vi "PH_Beckhoff-16BB.declare digital OutputTags.vi"(2 "Racktype":string, 3 "Digital Outputs to be inverted [#s separated by ::]":string, 4 "Instance Name":string="<Instance Name>") -> (0 "Digital Outputs":T1, 1 "Description":string)   [LabVIEW 2014, in "PH_Beckhoff-16BB.lvlib"]
uses:
  PH_Beckhoff-16BB.lvlib
  PH_Beckhoff/PH_Beckhoff.Digital Outputs.ctl
  PH_Beckhoff/PH_Beckhoff.lvlib
  PH_Beckhoff_Common/PH_Beckhoff_Common.lvlib
panel:
  out "Right Size?":bool
  # "Let this VI run to check the size!"
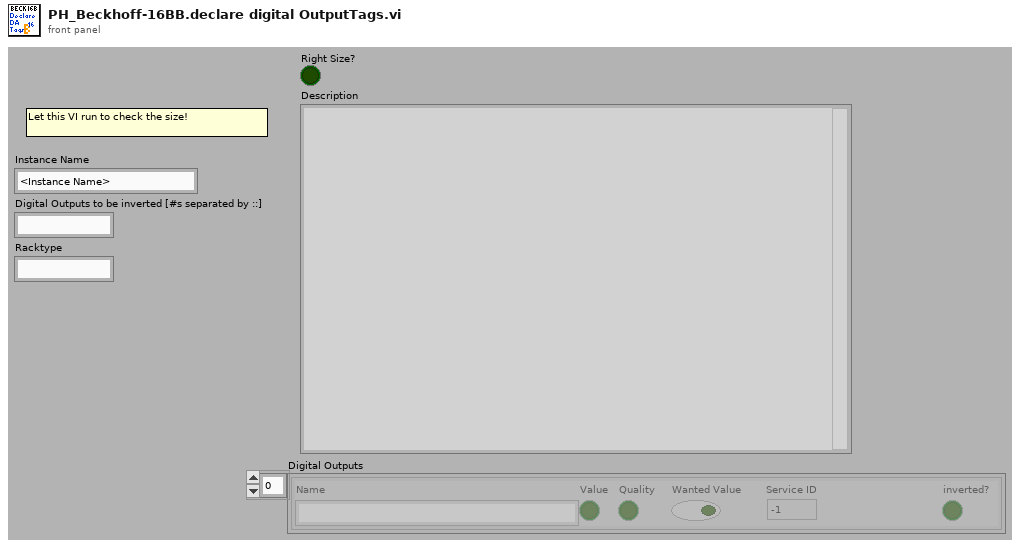
[diagram p1: front panel]
types:
  T1 = typedef "PH_Beckhoff.lvlib/PH_Beckhoff.Digital Outputs.ctl" = cluster{"Name":string, "Value":bool, "Quality":bool, "Wanted Value":bool, "Service ID":i32, "inverted?":bool}[]
  T2 = cluster{"Name":string, "Value":bool, "Quality":bool, "Wanted Value":bool, "Service ID":i32, "inverted?":bool}
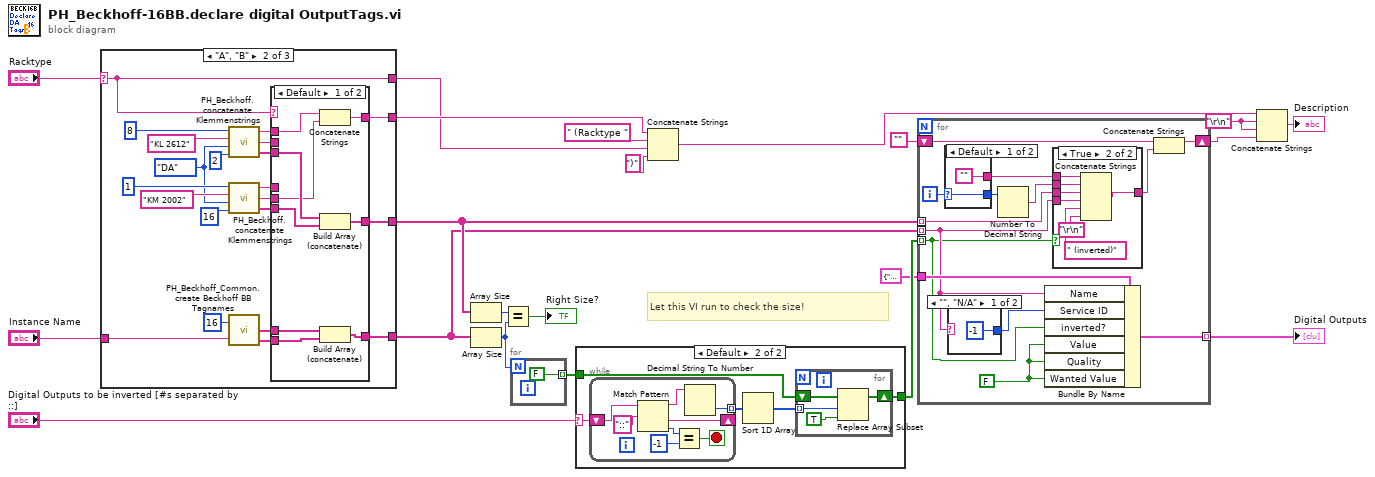
[diagram p0: block diagram]
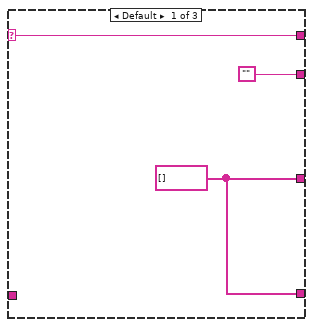
[diagram p2: hidden frame]
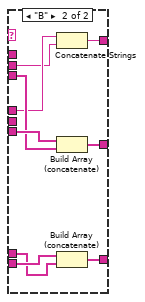
[diagram p3: hidden frame]
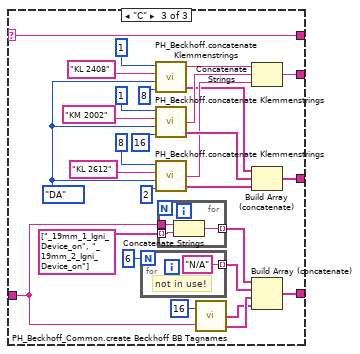
[diagram p4: hidden frame]
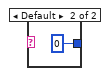
[diagram p6: hidden frame]
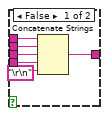
[diagram p7: hidden frame]
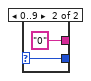
[diagram p8: hidden frame]
diagram:
  w21 = "\r\n"
  # "Let this VI run to check the size!"
  n1 = case shown="\"A\", \"B\"" "Racktype" {
    selector: "Racktype" -> [w24 w25 w77]
    tunnel: "Instance Name" -> [_ w35 w65]
    tunnel: [w22 w28 w80] -> w3
    tunnel: [w22 w27 w79] -> w4
    tunnel: ["" w26 w78] -> w10
    tunnel: [w24 w25 w77] -> w6
    frame Default {
      w22 = string[] []
    }
    frame "A", "B" {
      w39 = enum16{"AE", "AA", "DE", "DA"}."DA" ("Type")
      n2 = call "PH_Beckhoff.concatenate Klemmenstrings.vi"("# of In- or Outputs"=2, "Type"=w39, "Klemmenname"="KL 2612", "Quantity"=8 ("size(s)")) -> ("concatenated string array"=w34:string[], "\"and <Quantity> x <Klemmenname>\""=w32:string, "\"<Type>: <Quantity> x <Klemmenname>\""=w30:string)
      n3 = call "PH_Beckhoff.concatenate Klemmenstrings.vi"("# of In- or Outputs"=16, "Type"=w39, "Klemmenname"="KM 2002", "Quantity"=1 ("size(s)")) -> ("concatenated string array"=w33:string[], "\"and <Quantity> x <Klemmenname>\""=w29:string, "\"<Type>: <Quantity> x <Klemmenname>\""=w31:string)
      n4 = call "PH_Beckhoff_Common.create Beckhoff BB Tagnames.vi"("#"=16, "Instance Name"=w35) -> ("move-in-Tags"=w37:string[], "move-Tags"=w38:string[])  [unwired: 1 out]
      n5 = case shown="Default" w25 {
        tunnel: w38 -> [w54 w62]
        tunnel: w37 -> [w53 w61]
        tunnel: [w52 w63] -> w28
        tunnel: w34 -> [w49 w58]
        tunnel: w33 -> [w48 w59]
        tunnel: [w51 w60] -> w27
        tunnel: w32 -> [_ w55]
        tunnel: w31 -> [_ w56]
        tunnel: [w50 w57] -> w26
        tunnel: w30 -> [w47 _]
        tunnel: w29 -> [w46 _]
        frame Default {
          n6 = Concatenate Strings(w47, w46) -> (w50:string)
          n7 = Build Array (concatenate)(w49, w48) -> (w51:string[])
          n8 = Build Array (concatenate)(w53, w54) -> (w52:string[])
        }
        frame "B" {
          n9 = Concatenate Strings(w56, w55) -> (w57:string)
          n10 = Build Array (concatenate)(w59, w58) -> (w60:string[])
          n11 = Build Array (concatenate)(w62, w61) -> (w63:string[])
        }
      }
    }
    frame "C" {
      w70 = enum16{"AE", "AA", "DE", "DA"}."DA" ("Type")
      n12 = for {
        N: 6 -> [_]
        tunnel: ["N/A" ("string")] -> w67 mode=indexing
        # "not in use!"
      }
      n13 = call "PH_Beckhoff.concatenate Klemmenstrings.vi"("# of In- or Outputs"=8, "Type"=w70, "Klemmenname"="KL 2408", "Quantity"=1 ("size(s)")) -> ("concatenated string array"=w69:string[], "\"<Type>: <Quantity> x <Klemmenname>\""=w71:string)  [unwired: 1 out]
      n14 = call "PH_Beckhoff.concatenate Klemmenstrings.vi"("# of In- or Outputs"=16, "Type"=w70, "Klemmenname"="KM 2002", "Quantity"=1 ("size(s)")) -> ("concatenated string array"=w82:string[], "\"and <Quantity> x <Klemmenname>\""=w75:string)  [unwired: 1 out]
      n15 = call "PH_Beckhoff.concatenate Klemmenstrings.vi"("# of In- or Outputs"=2, "Type"=w70, "Klemmenname"="KL 2612", "Quantity"=8 ("size(s)")) -> ("concatenated string array"=w83:string[], "\"and <Quantity> x <Klemmenname>\""=w81:string)  [unwired: 1 out]
      n16 = for {
        tunnel: w65 -> [w94]
        tunnel: [w93] -> w66 mode=indexing
        tunnel: string[] ["_19mm_1_Igni_Device_on", "_19mm_2_Igni_Device_on"] -> [w92] mode=indexing
        n17 = Concatenate Strings(w94, w92) -> (w93:string)
      }
      n18 = call "PH_Beckhoff_Common.create Beckhoff BB Tagnames.vi"("#"=16, "Instance Name"=w65) -> ("move-in-Tags"=w76:string[], "move-Tags"=w85:string[])  [unwired: 1 out]
      n19 = Concatenate Strings(w71, w75, w81) -> (w78:string)
      n20 = Build Array (concatenate)(w69, w82, w83) -> (w79:string[])
      n21 = Build Array (concatenate)(w66, w67, w85, w76) -> (w80:string[])
    }
  }
  n22 = Array Size(array=w4) -> (size(s)=w19:i32)
  n23 = Array Size(array=w3) -> (size(s)=w14:i32)
  n24 = Equal?(x=w19, y=w14) -> (x = y?=→"Right Size?":bool)
  n25 = for {
    N: w14 -> [_]
    tunnel: [FALSE] -> w16 mode=indexing
  }
  n26 = case shown="Default" "Digital Outputs to be inverted [#s separated by ::]" {
    selector: "Digital Outputs to be inverted [#s separated by ::]" -> [_ w102]
    tunnel: w16 -> [w97 w99]
    tunnel: [w97 w98] -> w5
    frame "", "N/A" {
    }
    frame Default {
      n27 = while {
        shift-right: [w109] -> _
        shift-left: w102 -> [w114]
        tunnel: [w107] -> w101 mode=indexing
        stop <- w110 stop-if-true
        n28 = Match Pattern(string=w114, regular expression="::") -> (before substring=w108:string, after substring=w109:string, offset past match=w112:i32)  [unwired: 1 in, 1 out]
        n29 = Equal?(x=w112, y=-1) -> (x = y?=w110:bool)
        n30 = Decimal String To Number(string=w108) -> (number=w107:i32)  [unwired: 2 in, 1 out]
      }
      n31 = Sort 1D Array(array=w101) -> (sorted array=w100:i32[])
      n32 = for {
        tunnel: w100 -> [w104] mode=indexing
        shift-right: [w105] -> w98
        shift-left: w99 -> [w106]
        n33 = Replace Array Subset(array=w106, new element=TRUE ("new element/subarray"), index=w104) -> (w105:bool[])
      }
    }
  }
  n34 = Concatenate Strings(w10, " (Racktype " ("string"), w6, ")" ("string")) -> (w9:string)
  n35 = for {
    tunnel: w3 -> [w119] mode=indexing
    tunnel: w4 -> [w124] mode=indexing
    shift-right: [w122] -> w13
    shift-left: "" -> [w121]
    tunnel: w5 -> [w117] mode=indexing
    tunnel: T2 {"Name"="", "Value"=FALSE, "Quality"=FALSE, "Wanted Value"=FALSE, "Service ID"=0, "inverted?"=FALSE} ("Digital Output Value") -> [w120]
    tunnel: [w115] -> w1 mode=indexing
    i -> [w128]
    w116 = FALSE ("Quality")
    n36 = case shown="Default" w128 {
      selector: w128 -> [w144 w147]
      tunnel: [w144 w147] -> w127
      tunnel: ["" "0"] -> w126
      frame Default {
      }
      frame 0..9 {
      }
    }
    n37 = case shown="\"\", \"N/A\"" w119 {
      tunnel: [-1 0] -> w118
      frame "", "N/A" {
      }
      frame Default {
      }
    }
    n38 = Number To Decimal String(number=w127) -> (decimal integer string=w125:string)  [unwired: 1 in]
    n39 = Bundle By Name(cluster=w120, "Name"=w119, "Service ID"=w118, "inverted?"=w117, "Value"=w116, "Quality"=w116, "Wanted Value"=w116) -> (w115:T2)
    n40 = case shown="True" w117 {
      tunnel: w126 -> [w136 w143]
      tunnel: w125 -> [w135 w142]
      tunnel: w124 -> [w134 w141]
      tunnel: w119 -> [w133 w140]
      tunnel: [w131 w138] -> w123
      frame False {
        n41 = Concatenate Strings(w136, w135, w134, w133, "\r\n") -> (w131:string)
      }
      frame True {
        n42 = Concatenate Strings(w143, w142, w141, w140, " (inverted)", "\r\n") -> (w138:string)
      }
    }
    n43 = Concatenate Strings(w121, w123) -> (w122:string)
  }
  "Digital Outputs" <- w1
  n44 = Concatenate Strings(w9, w21, w21, w13) -> (→"Description":string)
